vi "creator.vi"() -> ()   [LabVIEW 2010]
uses:
  common/classes/ErrorController/ErrorController/ErrorController.lvclass
  common/clusters/plugin_specification.ctl
  HelioWizardDL101109/wizard_cluster.ctl
  <vilib>/Platform/browser.llb/Open URL in Default Browser (string).vi
  common/classes/ErrorController/ErrorController/class_data.vi
panel:
  out "error handler loaded?":bool
  in  "deleteButton":bool
  in  "downButton":bool
  in  "upButton":bool
  in  "steps":i32(listbox)
  in  "addButton":bool
  in  "component class path":path
  in  "configuration name":string
  # "Wizard Creator"
  # "New step"
  # "Procedure"
  # "1. Enter the class file path of a HelioScan component to be configured.\n\n2. Enter the name of the configuration file to be created (without \".xml\" ending).\n\n3. Press the add button. A step will be added accordingly to the list of steps on the right.\n\n4. You can change the sequence of steps using the \"Move up\" and \"Move down\" buttons. You can also delete steps if required.\n\n5. Repeat steps 1-4 until you are finished. \n\n6. Reorder the components in order of inheritance. Then select File > Save as...\n\n7. Quit the wizard via File > Exit."
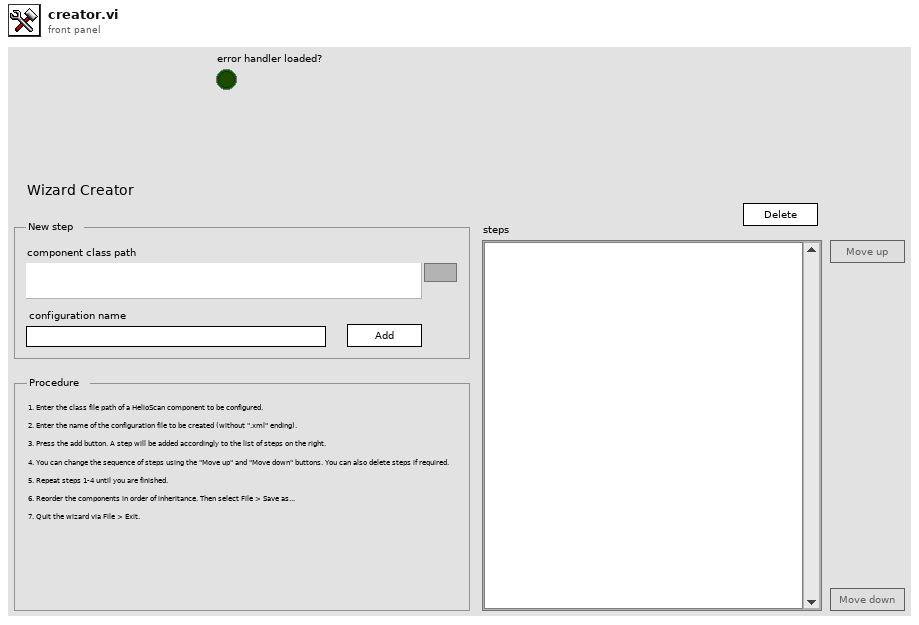
[diagram p1: front panel]
types:
  T1 = typedef "plugin_specification.ctl" = cluster{"class path":string, "configuration":string, "label":string, "settings name":string}
  T2 = enum8{"Enabled", "Disabled", "Disabled and Grayed Out"}
  T3 = typedef "wizard_cluster.ctl" = cluster{"step":T1[]}
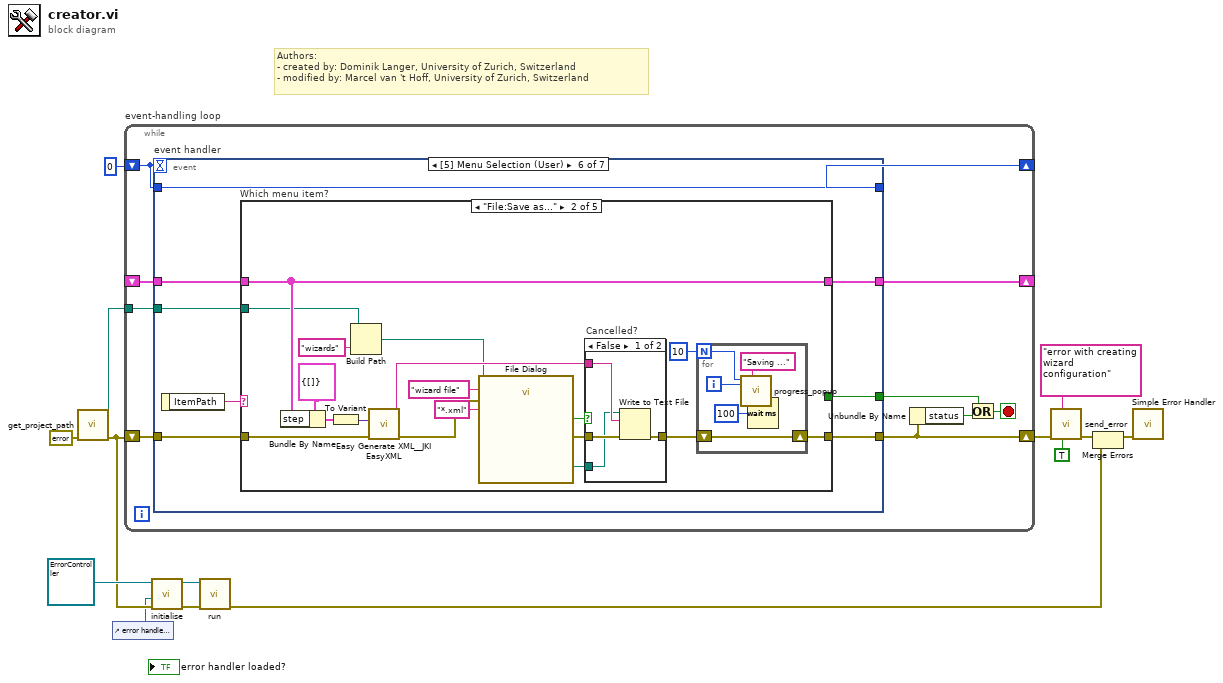
[diagram p0: block diagram]
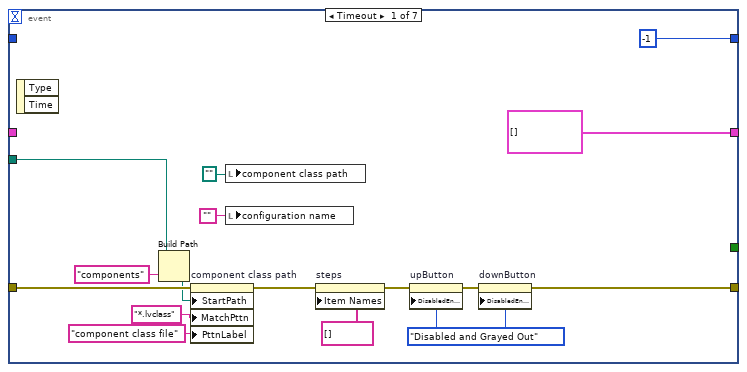
[diagram p2: hidden frame]
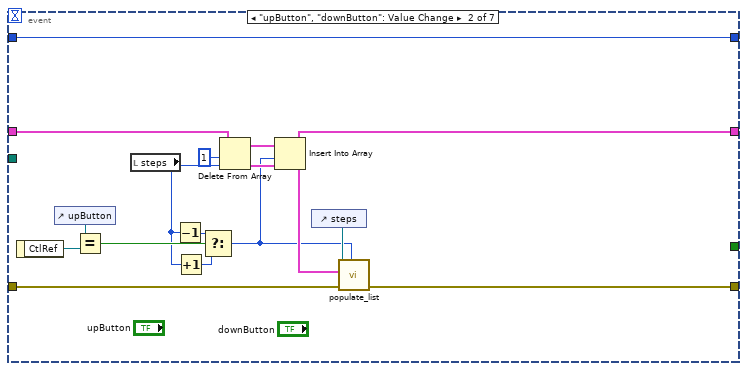
[diagram p3: hidden frame]
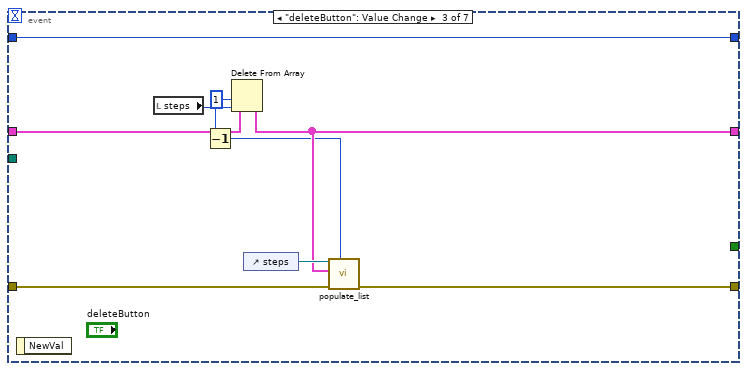
[diagram p4: hidden frame]
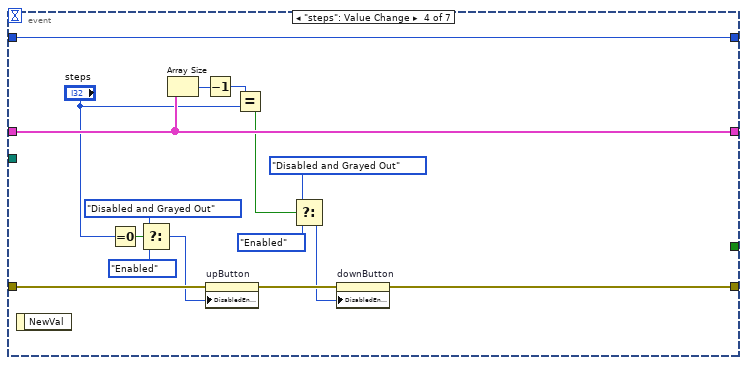
[diagram p5: hidden frame]
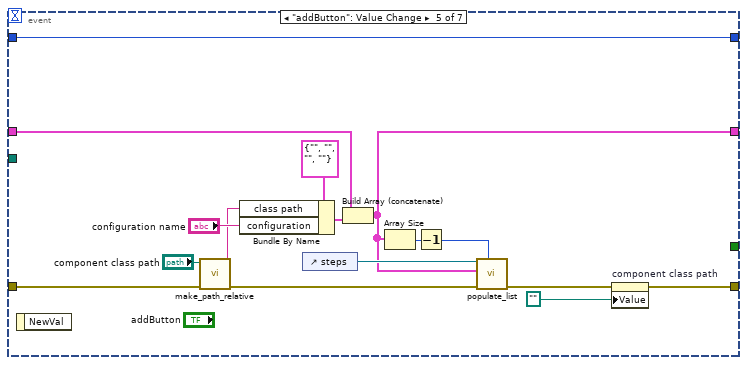
[diagram p6: hidden frame]
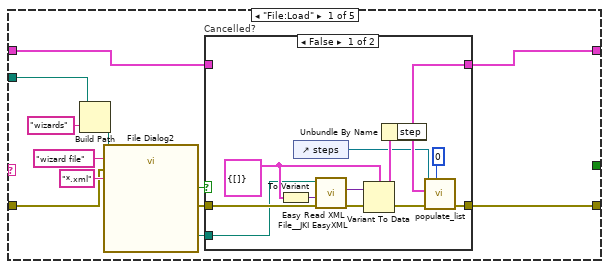
[diagram p7: hidden frame]
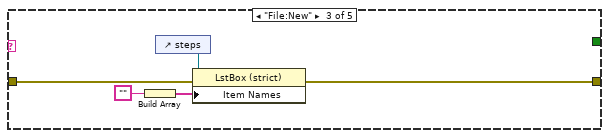
[diagram p10: hidden frame]
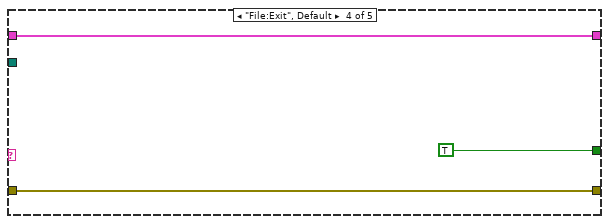
[diagram p11: hidden frame]
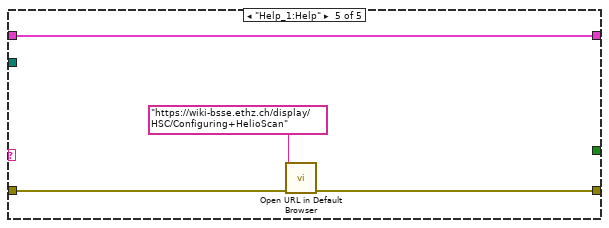
[diagram p12: hidden frame]
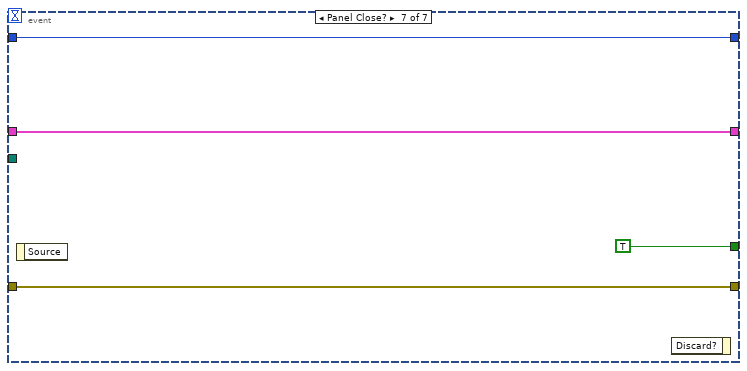
[diagram p13: hidden frame]
diagram:
  # "Authors: \n- created by: Dominik Langer, University of Zurich, Switzerland\n- modified by: Marcel van 't Hoff, University of Zurich, Switzerland"
  n1 = call "get_project_path.vi"("error in (no error)"=errorcluster {"status"=FALSE, "code"=0, "source"=""}) -> ("error out"=w10:errorcluster, "helioscan path"=w13:path)  [unwired: 9 in]
  n2 = control-ref of="error handler loaded?"() -> (w7:refnum<vi>)
  n3 = while "event-handling loop" {
    shift-right: [w23] -> w4
    shift-left: w10 -> [w24]
    shift-right: [w16] -> _
    shift-left: _ -> [w19]
    shift-right: [w17] -> _
    shift-left: 0 -> [w18]
    tunnel: w13 -> [w15]
    stop <- w20 stop-if-true
    n4 = event "event handler" shown="[5] Menu Selection (User)" {
      selector: _ -> [_ _ _ _ _ _ _]
      dyn-events: _ -> [_ _ _ _ _ _ _]
      timeout: w18 -> [_ _ _ _ _ _ _]
      tunnel: w24 -> [w35 w42 w60 w77 w92 w102 w174]
      tunnel: [w26 w51 w57 w74 w83 w101 w174] -> w23
      tunnel: [_ _ _ _ _ w100 TRUE] -> w21
      tunnel: w19 -> [_ w52 w64 w70 w87 w99 w172]
      tunnel: [-1 w56 w65 w81 w96 w104 w173] -> w17
      tunnel: w18 -> [_ w56 w65 w81 w96 w104 w173]
      tunnel: [T1[] [] w50 w61 w70 w86 w98 w172] -> w16
      tunnel: w15 -> [w32 _ _ _ _ w97 _]
      event Timeout {
        w25 = T2."Disabled and Grayed Out" ("Disabled")
        n5 = event-data() -> ()  [unwired: 1 in, 2 out]
        n6 = Build Path(base path=w32, name or relative path="components") -> (appended path=w31:path)
        n7 = property on="component class path" class="Path"(error in=w35, "StartPath"=w31, "MatchPttn"="*.lvclass" ("Browse Options:Match Pattern"), "PttnLabel"="component class file" ("Browse Options:Pattern Label")) -> (error out=w34:errorcluster)  [unwired: 1 in, 1 out]
        n8 = local write "component class path"(path "") -> ()
        n9 = local write "configuration name"("") -> ()
        n10 = property on="steps" class="LstBox (strict)"(error in=w34, "Item Names"=string[] []) -> (error out=w28:errorcluster)  [unwired: 1 in, 1 out]
        n11 = property on="upButton" class="Bool"(error in=w28, "DisabledEnum"=w25) -> (error out=w27:errorcluster)  [unwired: 1 in, 1 out]
        n12 = property on="downButton" class="Bool"(error in=w27, "DisabledEnum"=w25) -> (error out=w26:errorcluster)  [unwired: 1 in, 1 out]
      }
      event "upButton", "downButton": Value Change {
        n13 = event-data() -> ("CtlRef"=w48:refnum<vi>)  [unwired: 1 in]
        n14 = control-ref of="upButton"() -> (w47:refnum<vi>)
        n15 = Equal?(x=w47, y=w48) -> (x = y?=w46:bool)
        n16 = local read "steps"() -> (w44:i32)
        n17 = Decrement(x=w44) -> (x-1=w45:i32)
        n18 = Increment(x=w44) -> (x+1=w43:i32)
        n19 = Select(t=w45, s=w46, f=w43) -> (s? t:f=w41:i32)
        n20 = Delete From Array(array=w52, length=1, index=w44) -> (deleted portion=w53:T1[], array with subset deleted=w54:T1[])
        n21 = Insert Into Array(array=w54, index=w41, new element=w53) -> (w50:T1[])
        n22 = control-ref of="steps"() -> (w49:refnum<vi>)
        n23 = call "populate_list.vi"("selected item (index)"=w41, "error in (no error)"=w42, "steps"=w50, "list ctrl reference"=w49) -> ("error out"=w51:errorcluster)  [unwired: 7 in]
      }
      event "deleteButton": Value Change {
        w59 = 1 ("length")
        n24 = event-data() -> ()  [unwired: 1 in, 1 out]
        n25 = local read "steps"() -> (w63:i32)
        n26 = Decrement(x=w59) -> (x-1=w58:i32)
        n27 = Delete From Array(array=w64, length=w59, index=w63) -> (array with subset deleted=w61:T1[])  [unwired: 1 out]
        n28 = control-ref of="steps"() -> (w62:refnum<vi>)
        n29 = call "populate_list.vi"("selected item (index)"=w58, "error in (no error)"=w60, "steps"=w61, "list ctrl reference"=w62) -> ("error out"=w57:errorcluster)  [unwired: 7 in]
      }
      event "steps": Value Change {
        n30 = event-data() -> ()  [unwired: 1 in, 1 out]
        n31 = Equal To 0?(x="steps") -> (x = 0?=w80:bool)
        n32 = Select(t=T2."Disabled and Grayed Out" ("Disabled"), s=w80, f=T2."Enabled" ("Disabled")) -> (s? t:f=w76:T2)
        n33 = Array Size(array=w70) -> (size(s)=w69:i32)
        n34 = Decrement(x=w69) -> (x-1=w68:i32)
        n35 = property on="upButton" class="Bool"(error in=w77, "DisabledEnum"=w76) -> (error out=w75:errorcluster)  [unwired: 1 in, 1 out]
        n36 = Equal?(x=w68, y="steps") -> (x = y?=w66:bool)
        n37 = Select(t=T2."Disabled and Grayed Out" ("Disabled"), s=w66, f=T2."Enabled" ("Disabled")) -> (s? t:f=w72:T2)
        n38 = property on="downButton" class="Bool"(error in=w75, "DisabledEnum"=w72) -> (error out=w74:errorcluster)  [unwired: 1 in, 1 out]
      }
      event "addButton": Value Change {
        n39 = event-data() -> ()  [unwired: 1 in, 1 out]
        n40 = call "make_path_relative.vi"("error in (no error)"=w92, "absolute path"="component class path") -> ("error out"=w91:errorcluster, "relative path"=w89:string)  [unwired: 8 in]
        n41 = Bundle By Name(cluster=T1 {"class path"="", "configuration"="", "label"="", "settings name"=""} ("component specification"), "class path"=w89, "configuration"="configuration name") -> (w88:T1)
        n42 = control-ref of="steps"() -> (w95:refnum<vi>)
        n43 = Build Array (concatenate)(w87, w88) -> (w86:T1[])
        n44 = Array Size(array=w86) -> (size(s)=w85:i32)
        n45 = Decrement(x=w85) -> ()  [unwired: 1 out]
        n46 = call "populate_list.vi"("selected item (index)"=w85, "error in (no error)"=w91, "steps"=w86, "list ctrl reference"=w95) -> ("error out"=w84:errorcluster)  [unwired: 7 in]
        n47 = property on="component class path" class="Path"(error in=w84, "Value"=path "") -> (error out=w83:errorcluster)  [unwired: 1 in, 1 out]
      }
      event Menu Selection (User) {
        n48 = event-data() -> ("ItemPath"=w103:string)  [unwired: 1 in]
        n49 = case "Which menu item?" shown="\"File:Save as...\"" w103 {
          tunnel: w102 -> [w109 w136 w162 w166 w168]
          tunnel: [w116 w132 w163 w166 w167] -> w101
          tunnel: [_ _ _ TRUE _] -> w100
          tunnel: w99 -> [w105 w137 _ w165 w170]
          tunnel: [w115 w137 _ w165 w170] -> w98
          tunnel: w97 -> [w110 w135 _ _ _]
          frame "File:Load" {
            n50 = Build Path(base path=w110, name or relative path="wizards") -> (appended path=w111:path)
            n51 = call "File Dialog2"("start path"=w111, "error in"=w109, "pattern (all files)"="*.xml", "pattern label"="wizard file") -> ("selected path"=w107:path, "cancelled"=w106:bool, "error out"=w108:errorcluster)  [unwired: 8 in, 1 out]
            n52 = case "Cancelled?" shown="False" w106 {
              tunnel: [w120 w130] -> w116
              tunnel: [w119 w129] -> w115
              tunnel: w108 -> [w123 w130]
              tunnel: w107 -> [w122 _]
              tunnel: w105 -> [_ w129]
              frame False {
                w125 = T3 {"step"=[]}
                n53 = To Variant(anything=w125) -> (Variant=w128:variant)
                n54 = control-ref of="steps"() -> (w118:refnum<vi>)
                n55 = call <vilib>:"Easy Read XML File__JKI EasyXML.vi"("error in (no error)"=w123, "LabVIEW Data (Type)"=w128, "XML File Path"=w122) -> ("error out"=w127:errorcluster, "LabVIEW Data"=w126:variant)  [unwired: 6 in, 1 out]
                n56 = Variant To Data(error in=w127, Variant=w126, type=w125) -> (error out=w121:errorcluster, data=w124:T3)
                n57 = Unbundle By Name(w124) -> ("step"=w119:T1[])
                n58 = call "populate_list.vi"("selected item (index)"=0, "error in (no error)"=w121, "steps"=w119, "list ctrl reference"=w118) -> ("error out"=w120:errorcluster)  [unwired: 7 in]
              }
              frame True {
              }
            }
          }
          frame "File:Save as..." {
            n59 = Bundle By Name(cluster=T3 {"step"=[]} ("wizard"), "step"=w137) -> (w139:T3)
            n60 = To Variant(anything=w139) -> (Variant=w138:variant)
            n61 = Build Path(base path=w135, name or relative path="wizards") -> (appended path=w134:path)
            n62 = call <vilib>:"Easy Generate XML__JKI EasyXML.vi"("error in (no error)"=w136, "LabVIEW Data"=w138) -> ("error out"=w141:errorcluster, "XML String"=w140:string)  [unwired: 1 in, 7 out]
            n63 = call "File Dialog"("start path"=w134, "error in"=w141, "pattern (all files)"="*.xml", "pattern label"="wizard file") -> ("selected path"=w145:path, "cancelled"=w146:bool, "error out"=w142:errorcluster)  [unwired: 8 in, 1 out]
            n64 = case "Cancelled?" shown="False" w146 {
              tunnel: w140 -> [w157 _]
              tunnel: [w156 w158] -> w131
              tunnel: w142 -> [w155 w158]
              tunnel: w145 -> [w154 _]
              frame False {
                n65 = Write to Text File(file (use dialog)=w154, text=w157, error in=w155) -> (error out=w156:errorcluster)  [unwired: 3 out]
              }
              frame True {
              }
            }
            n66 = for {
              N: 10 -> [w152]
              shift-right: [w149] -> w132
              shift-left: w131 -> [w149]
              i -> [w153]
              n67 = call "progress_popup.vi"("custom text"="Saving ...", "current"=w153, "total"=w152) -> ()  [unwired: 9 in]
              n68 = Wait (ms)(milliseconds to wait=u32 100) -> ()  [unwired: 1 out]
            }
          }
          frame "File:New" {
            n69 = Build Array("") -> (w159:string[])
            n70 = control-ref of="steps"() -> (w161:refnum<vi>)
            n71 = property class="LstBox (strict)"(reference=w161, error in=w162, "Item Names"=w159) -> (error out=w163:errorcluster)  [unwired: 1 out]
          }
          frame "File:Exit", Default {
          }
          frame "Help_1:Help" {
            n72 = call-poly <vilib>:"Open URL in Default Browser.vi"("error in (no error)"=w168, "URL"="https://wiki-bsse.ethz.ch/display/HSC/Configuring+HelioScan") -> ("error out"=w167:errorcluster)  [unwired: 4 in, 1 out]
          }
        }
      }
      event Panel Close? {
        n73 = event-data() -> ()  [unwired: 1 in, 1 out]
        n74 = event-data() -> ()  [unwired: 2 in, 1 out]
      }
    }
    n75 = Unbundle By Name(w23) -> ("status"=w22:bool)
    n76 = Or(x=w21, y=w22) -> (x .or. y?=w20:bool)
  }
  n77 = call-dynamic "initialise.vi"("error in (no error)"=w10, "error boolean"=w7, "ErrorController in"=refnum<class "ErrorController.lvclass"> refnum) -> ("error out"=w9:errorcluster, "ErrorController out"=w8:refnum<class "ErrorController.lvclass">)  [unwired: 7 in]
  n78 = call "run.vi"("error in (no error)"=w9, "ErrorController in"=w8) -> ("error out"=w5:errorcluster)  [unwired: 8 in, 1 out]
  n79 = call "send_error.vi"("last error? (F)"=TRUE, "additional message"="error with creating wizard configuration", "error in (no error)"=w4) -> ("error out"=w3:errorcluster)  [unwired: 8 in]
  n80 = Merge Errors(w3, w5) -> (w6:errorcluster)
  n81 = call <vilib>:"Simple Error Handler.vi"("error in (no error)"=w6) -> ()  [unwired: 4 in, 5 out]
